vi "IO Process GLB.vi"() -> ()   [LabVIEW 2019]
panel:
  out "IOProcess Root Path":path
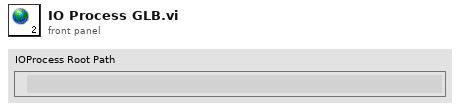
[diagram p1: front panel]
diagram:
